vi "Read_Wrap.vi"(8 "error in (no error)":errorcluster, 11 "Var_DBL in":refnum<class "Var_CPLX_SGL.lvclass">) -> (0 "error out":errorcluster, 2 "Value":T1, 3 "Var_DBL out":refnum<class "Var_CPLX_SGL.lvclass">)   [LabVIEW 2021, in "Var_CPLX_SGL.lvclass"]
uses:
  Var_CPLX_SGL.lvclass
  Var_CPLX_SGL.lvclass/Var_CPLX_SGL.ctl
  Type.ctl
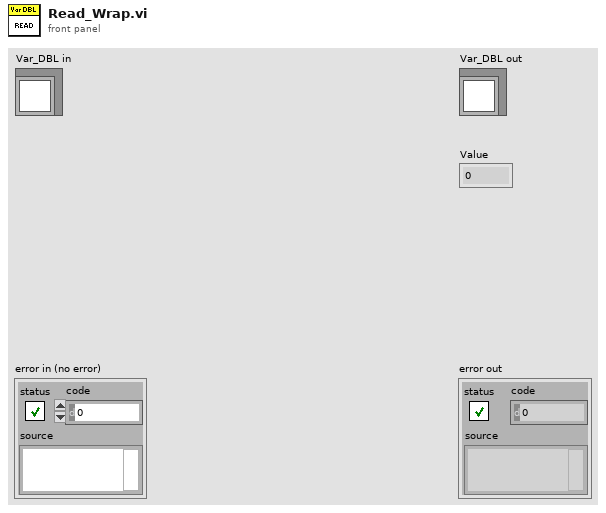
[diagram p1: front panel]
types:
  T1 = typedef "Var_CPLX_SGL.lvclass/Type.ctl" = dbl
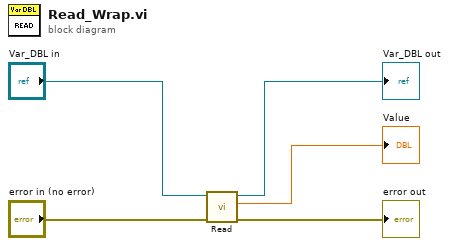
[diagram p0: block diagram]
diagram:
  n1 = call-dynamic "Read.vi"("error in (no error)"="error in (no error)", "Numeric in"="Var_DBL in") -> ("error out"=→"error out":errorcluster, "Numeric"=→"Value":T1, "Numeric out"=→"Var_DBL out":refnum<class "Var_CPLX_SGL.lvclass">)  [unwired: 7 in]
